vi "Time Check2.vi"(7 "error in":errorcluster, 8 "Elapsed Time":dbl, 9 "Last Time Stamp":dbl, 10 "Time Target":dbl) -> (0 "error out":errorcluster, 1 "New Elapsed Time":dbl, 2 "New Time Stamp":dbl, 3 "Status":cluster{"Running":bool, "Done":bool})   [LabVIEW 2014]
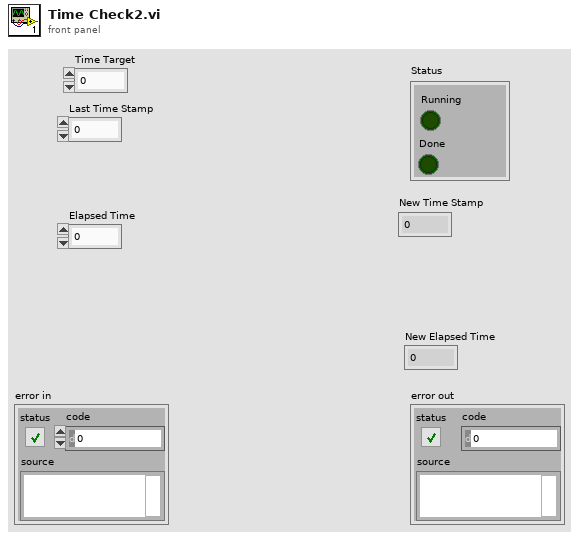
[diagram p1: front panel]
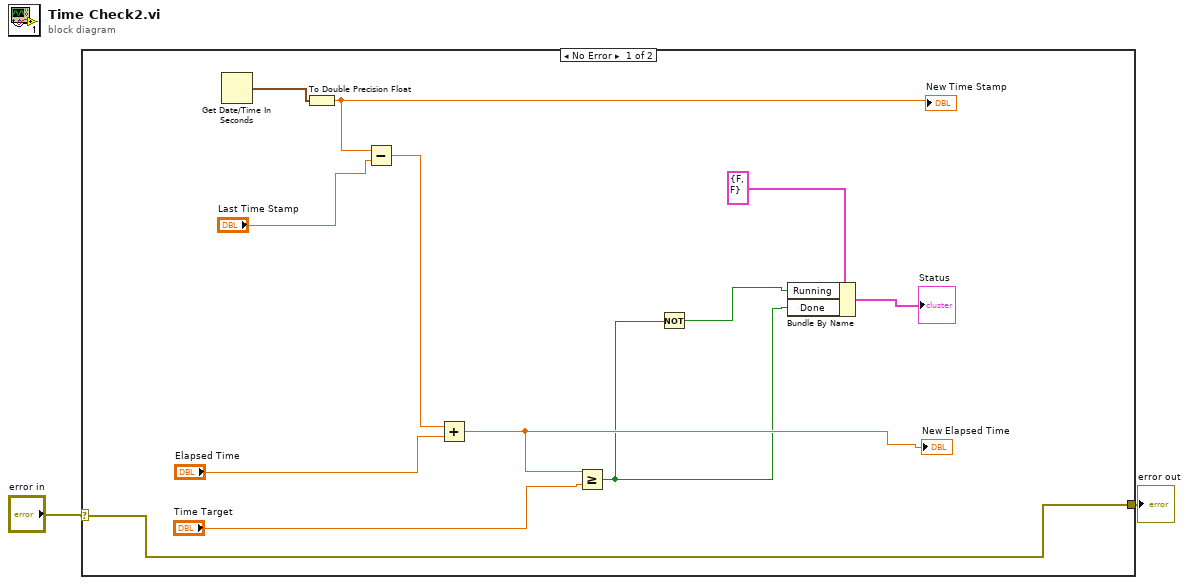
[diagram p0: block diagram]
diagram:
  n1 = case shown="No Error" "error in" {
    selector: "error in" -> [w4 w15]
    tunnel: [w4 w15] -> w1
    frame No Error {
      n2 = Get Date/Time In Seconds() -> (seconds since 1Jan1904=w14:timestamp)
      n3 = To Double Precision Float(number=w14) -> (double precision float=w12:dbl)
      "New Time Stamp" <- w12
      n4 = Subtract(x=w12, y="Last Time Stamp") -> (x-y=w10:dbl)
      n5 = Add(x=w10, y="Elapsed Time") -> (x+y=w8:dbl)
      "New Elapsed Time" <- w8
      n6 = Greater Or Equal?(x=w8, y="Time Target") -> (x >= y?=w6:bool)
      n7 = Not(x=w6) -> (.not. x?=w5:bool)
      n8 = Bundle By Name(cluster=cluster{"Running":bool, "Done":bool} {"Running"=FALSE, "Done"=FALSE} ("Status 2"), "Running"=w5, "Done"=w6) -> (→"Status":cluster{"Running":bool, "Done":bool})
    }
    frame Error {
    }
  }
  "error out" <- w1
